vi "08_LOGfilewrite.vi"(9 "Counters":T1, 10 "output cluster":cluster{dbl, dbl, dbl}, 11 "refnum out":refnum<file>) -> ()   [LabVIEW 2017]
uses:
  <vilib>/Utility/error.llb/whitespace.ctl
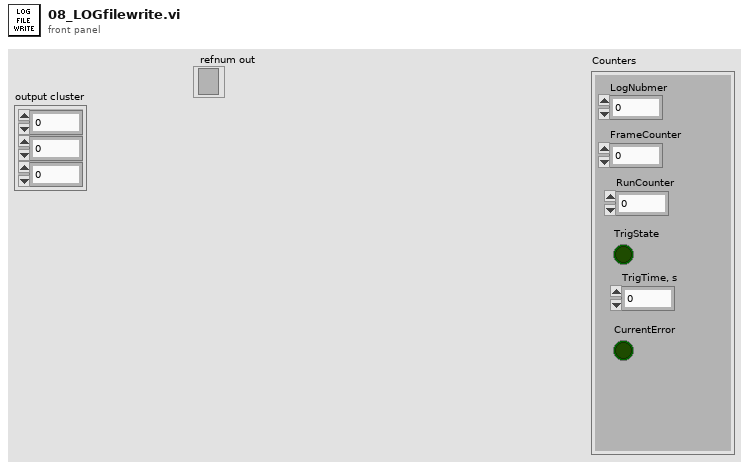
[diagram p1: front panel]
types:
  T1 = cluster{"LogNubmer":i32, "FrameCounter":i32, "RunCounter":u32, "TrigState":bool, "TrigTime, s":dbl, "CurrentError":bool}
  T2 = typedef "whitespace.ctl" = u16
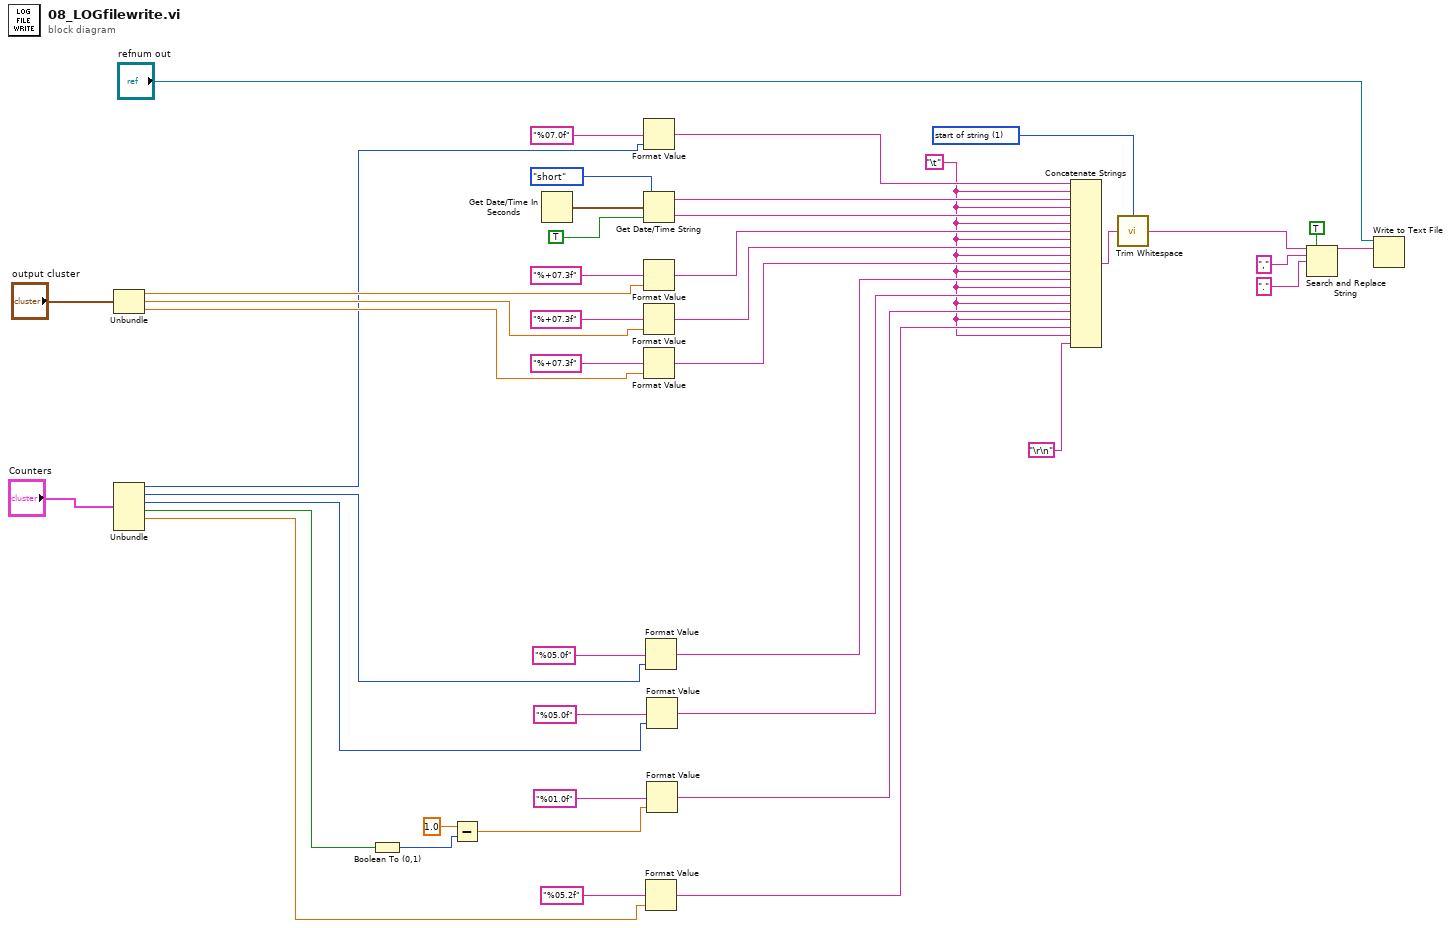
[diagram p0: block diagram]
diagram:
  w2 = "\t"
  w33 = T2 1 items=["both", "start of string", "end of string"] ("location (both)")
  n1 = Unbundle("output cluster") -> (w23:dbl, w22:dbl, w21:dbl)
  n2 = Unbundle("Counters") -> ("LogNubmer"=w17:i32, "FrameCounter"=w16:i32, "RunCounter"=w15:u32, "TrigState"=w8:bool, "TrigTime, s"=w10:dbl)  [unwired: 1 out]
  n3 = Boolean To (0,1)(Boolean=w8) -> (0, 1=w9:i16)
  n4 = Subtract(x=1.0, y=w9) -> (x-y=w12:dbl)
  n5 = Get Date/Time In Seconds() -> (seconds since 1Jan1904=w40:timestamp)
  n6 = Format Value(format string="%07.0f", value (0)=w17) -> (output string=w30:string)  [unwired: 1 in]
  n7 = Get Date/Time String(date format (0)=enum16{"short", "long", "abbreviated"}."short", seconds (now)=w40, want seconds? (F)=TRUE) -> (date string=w31:string, time string=w32:string)
  n8 = Format Value(format string="%+07.3f", value (0)=w23) -> (output string=w37:string)  [unwired: 1 in]
  n9 = Format Value(format string="%+07.3f", value (0)=w22) -> (output string=w36:string)  [unwired: 1 in]
  n10 = Format Value(format string="%+07.3f", value (0)=w21) -> (output string=w35:string)  [unwired: 1 in]
  n11 = Format Value(format string="%05.0f", value (0)=w16) -> (output string=w6:string)  [unwired: 1 in]
  n12 = Format Value(format string="%05.2f", value (0)=w10) -> (output string=w3:string)  [unwired: 1 in]
  n13 = Format Value(format string="%05.0f", value (0)=w15) -> (output string=w5:string)  [unwired: 1 in]
  n14 = Format Value(format string="%01.0f", value (0)=w12) -> (output string=w4:string)  [unwired: 1 in]
  n15 = Concatenate Strings(w30, w2, w31, w2, w32, w2, w37, w2, w36, w2, w35, w2, w6, w2, w5, w2, w4, w2, w3, w2, "\r\n") -> (w34:string)
  n16 = call <vilib>:"Trim Whitespace.vi"("string"=w34, "location (both)"=w33) -> ("trimmed string"=w26:string)
  n17 = Search and Replace String(replace all?=TRUE ("replace all? (F)"), input string=w26, search string=",", replace string="." ("replace string (\"\")")) -> (result string=w25:string)  [unwired: 4 in, 3 out]
  n18 = Write to Text File(file (use dialog)="refnum out", text=w25) -> ()  [unwired: 2 in, 3 out]
